vi "Get Size of Data from TD - Benchmark Map Collection of Fixed-size Value (String,Int32) - Should Perform in O(n)+O(1).vi"() -> ()   [LabVIEW 2017, in "Composition.Tests.lvlib"]
uses:
  Composition.Tests.lvlib
  <vilib>/addons/_JKI Toolkits/Caraya/classes/Assert/Assert Less_Variant.vi
  Composition/Composition.lvlib
  <vilib>/addons/_JKI Toolkits/Caraya/classes/Test/Test.lvclass
  <vilib>/addons/_JKI Toolkits/Caraya/classes/Assert/Assert.lvclass
panel:
  out "error out":errorcluster
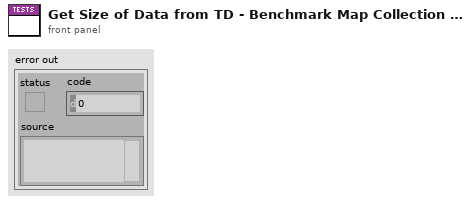
[diagram p1: front panel]
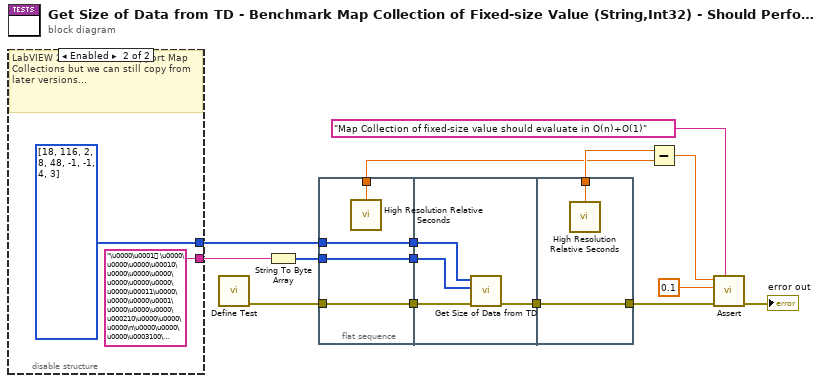
[diagram p0: block diagram]
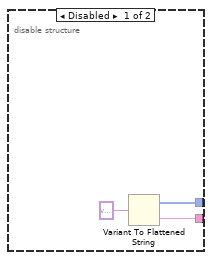
[diagram p2: hidden frame]
diagram:
  n1 = disable-structure shown="Enabled" {
    disable-tunnel: [w18 "\u0000\u0001 \u0000\u0000\u0000\u00010\u0000\u0000\u0000\u0000\u0000\u0000\u0000\u00011\u0000\u0000\u0000\u0001\u0000\u0000\u0000\u000210\u0000\u0000\u0000\n\u0000\u0000\u0000\u0003100\u0000\u0000\u0000d\u0000\u0000\u0000\u00041000\u0000\u0000\u0003è\u0000\u0000\u0000\u000510000\u0000\u0000'\u0010\u0000\u0000\u0000\u000510001\u0000\u0000'\u0011\u0000\u0000\u0000\u000510002\u0000\u0000'\u0012\u0000\u0000\u0000\u000510003\u0000\u0000'\u0013\u0000\u0000\u0000\u000510004\u0000\u0000'\u0014\u0000\u0000\u0000\u000510005\u0000\u0000'\u0015\u0000\u0000\u0000\u000510006\u0000\u0000'\u0016\u0000\u0000\u0000\u000510007\u0000\u0000'\u0017\u0000\u0000\u0000\u000510008\u0000\u0000'\u0018\u0000\u0000\u0000\u000510009\u0000\u0000'\u0019\u0000\u0000\u0000\u00041001\u0000\u0000\u0003é\u0000\u0000\u0000\u000510010\u0000\u0000'\u001a\u0000\u0000\u0000\u000510011\u0000\u0000'\u001b\u0000\u0000\u0000\u000510012\u0000\u0000'\u001c\u0000\u0000\u0000\u000510013\u0000\u0000'\u001d\u0000\u0000\u0000\u000510014\u0000\u0000'\u001e\u0000\u0000\u0000\u000510015\u0000\u0000'\u001f\u0000\u0000\u0000\u000510016\u0000\u0000' \u0000\u0000\u0000\u000510017\u0000\u0000'!\u0000\u0000\u0000\u000510018\u0000\u0000'\"\u0000\u0000\u0000\u000510019\u0000\u0000'#\u0000\u0000\u0000\u00041002\u0000\u0000\u0003ê\u0000\u0000\u0000\u000510020\u0000\u0000'$\u0000\u0000\u0000\u000510021\u0000\u0000'%\u0000\u0000\u0000\u000510022\u0000\u0000'&\u0000\u0000\u0000\u000510023\u0000\u0000''\u0000\u0000\u0000\u000510024\u0000\u0000'(\u0000\u0000\u0000\u000510025\u0000\u0000')\u0000\u0000\u0000\u000510026\u0000\u0000'*\u0000\u0000\u0000\u000510027\u0000\u0000'+\u0000\u0000\u0000\u000510028\u0000\u0000',\u0000\u0000\u0000\u000510029\u0000\u0000'-\u0000\u0000\u0000\u00041003\u0000\u0000\u0003ë\u0000\u0000\u0000\u000510030\u0000\u0000'.\u0000\u0000\u0000\u000510031\u0000\u0000'/\u0000\u0000\u0000\u000510032\u0000\u0000'0\u0000\u0000\u0000\u000510033\u0000\u0000'1\u0000\u0000\u0000\u000510034\u0000\u0000'2\u0000\u0000\u0000\u000510035\u0000\u0000'3\u0000\u0000\u0000\u000510036\u0000\u0000'4\u0000\u0000\u0000\u000510037\u0000\u0000'5\u0000\u0000\u0000\u000510038\u0000\u0000'6\u0000\u0000..." ("data string")] -> w1
    disable-tunnel: [w16 i16[] [18, 116, 2, 8, 48, -1, -1, 4, 3] ("Type Descriptor")] -> w2
    frame Disabled {
      n2 = Variant To Flattened String(Variant=variant) -> (data string=w18:string, 1:w16:i16[])
    }
    frame Enabled {
      # "LabVIEW 2017 does not support Map Collections but we can still copy from later versions..."
    }
  }
  n3 = call <vilib>:"Define Test.vi"() -> ("error out"=w14:errorcluster)  [unwired: 11 in]
  n4 = String To Byte Array(string=w1) -> (unsigned byte array=w15:u8[])
  n5 = flat-sequence {
    tunnel: w14 -> [w22]
    tunnel: w15 -> [w23]
    tunnel: w2 -> [w24]
    tunnel: [w24] -> w13
    tunnel: [w23] -> w12
    tunnel: [w22] -> w11
    tunnel: [w21] -> w9
    tunnel: w13 -> [w28]
    tunnel: w12 -> [w27]
    tunnel: w11 -> [w26]
    tunnel: [w25] -> w8
    tunnel: [w30] -> w10
    tunnel: [w29] -> w7
    tunnel: w8 -> [w29]
    frame #0 {
      n6 = call <vilib>:"High Resolution Relative Seconds.vi"() -> ("relative seconds"=w21:dbl)
    }
    frame #1 {
      n7 = call "Get Size of Data from TD.vi"("error in (no error)"=w26, "Data String"=w27, "Type Descriptor"=w28) -> ("error out"=w25:errorcluster)  [unwired: 7 in, 1 out]
    }
    frame #2 {
      n8 = call <vilib>:"High Resolution Relative Seconds.vi"() -> ("relative seconds"=w30:dbl)
    }
  }
  n9 = Subtract(x=w10, y=w9) -> (x-y=w6:dbl)
  n10 = call-poly <vilib>:"Assert.vi"("Label"="Map Collection of fixed-size value should evaluate in O(n)+O(1)", "error in (no error)"=w7, "Y"=0.1 ("x-y"), "X"=w6) -> ("error out"=→"error out":errorcluster)  [unwired: 7 in]
